vi "JL_Diag_Filter_Seq.vi"(0 "Filter by Count":bool, 5 "Fault Table Entries In":T2[](array[typedef]), 7 "Status":T1) -> (4 "Fault Table Entries Out":T2[](array[typedef]))   [LabVIEW 2018]
uses:
  Common/Diagnostics Decode/Type Defs/Diag_FaultSeqEntry.ctl
  Common/Diagnostics Decode/Type Defs/Diag_FaultTableStatus.ctl
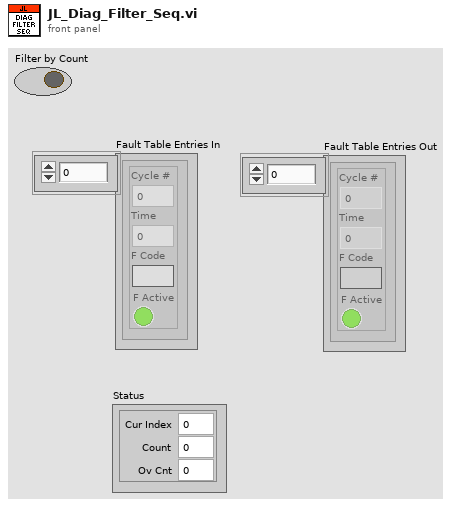
[diagram p1: front panel]
types:
  T1 = typedef "Diag_FaultTableStatus.ctl" = cluster{"Cur Index":u16, "Count":u16, "Ov Cnt":u16}
  T2 = typedef "Diag_FaultSeqEntry.ctl" = cluster{"Cycle #":u32, "Time":u32, "F Code":string, "F Active":bool}
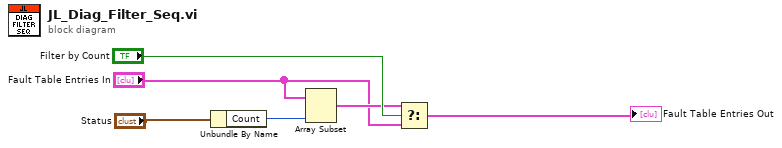
[diagram p0: block diagram]
diagram:
  n1 = Unbundle By Name("Status") -> ("Count"=w4:u16)
  n2 = Array Subset(array="Fault Table Entries In", length=w4) -> (w5:T2[])  [unwired: 1 in]
  n3 = Select(t=w5, s="Filter by Count", f="Fault Table Entries In") -> (s? t:f=→"Fault Table Entries Out":T2[])
